vi "RC_Init.vi"(8 "error in (no error)":errorcluster, 10 "Condition #":i32, 11 "Reward_Condition in":refnum<class "Reward_Condition.lvclass">) -> (0 "error out":errorcluster, 3 "Reward_Condition out":refnum<class "Reward_Condition.lvclass">)   [LabVIEW 2018, in "Tracker.lvlib" / "Reward_Condition.lvclass"]
uses:
  Reward_Condition.lvclass
  Reward_SubCondition/Reward_SubCondition.lvclass
  Reward_Condition.lvclass/Reward_Condition.ctl
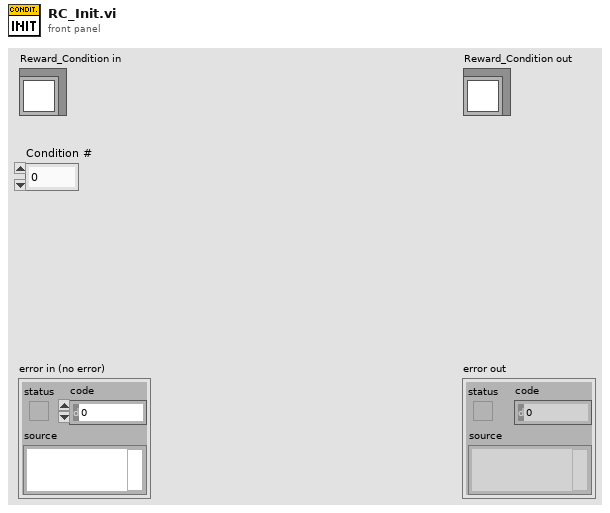
[diagram p1: front panel]
types:
  T1 = enum16{"None", "Port 1", "Port 2", "Port 3", "Port 4"}
  T2 = enum16{"None", "TTL pulse", "TTL trigger", "Air puff", "Liquid reward"}
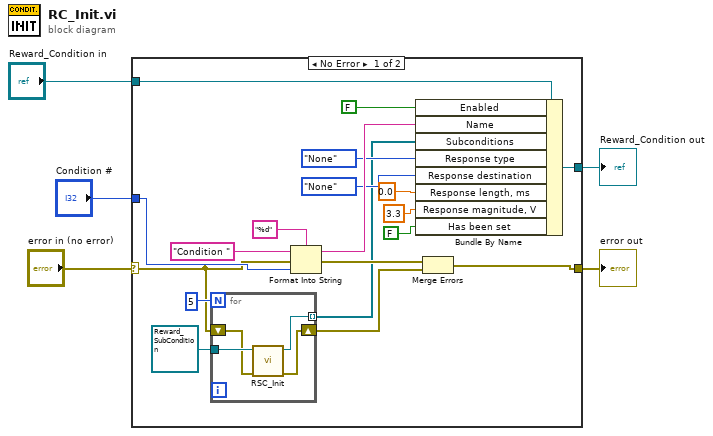
[diagram p0: block diagram]
diagram:
  n1 = case shown="No Error" "error in (no error)" {
    selector: "error in (no error)" -> [w8 w30]
    tunnel: [w7 w30] -> w4
    tunnel: [w23 w29] -> w2
    tunnel: "Reward_Condition in" -> [w24 w29]
    tunnel: "Condition #" -> [w20 _]
    frame No Error {
      n2 = for {
        N: 5 -> [_]
        tunnel: refnum<class "Reward_SubCondition.lvclass"> refnum ("Tracker.lvlib:Reward_SubCondition.lvclass") -> [w28]
        tunnel: [w27] -> w9 mode=indexing
        shift-right: [w25] -> w6
        shift-left: w8 -> [w26]
        n3 = call "RSC_Init.vi"("error in (no error)"=w26, "Reward_SubCondition in"=w28) -> ("error out"=w25:errorcluster, "Reward_SubCondition out"=w27:refnum<class "Reward_SubCondition.lvclass">)  [unwired: 8 in]
      }
      n4 = Format Into String(format string="%d", initial string="Condition ", error in=w8, w20) -> (resulting string=w19:string, error out=w13:errorcluster)
      n5 = Bundle By Name(cluster=w24, "Enabled"=FALSE, "Name"=w19, "Subconditions"=w9, "Response type"=T2."None", "Response destination"=T1."None", "Response length, ms"=0.0, "Response magnitude, V"=3.3, "Has been set"=FALSE) -> (w23:refnum<class "Reward_Condition.lvclass">)
      n6 = Merge Errors(w13, w6) -> (w7:errorcluster)
    }
    frame Error {
    }
  }
  "error out" <- w4
  "Reward_Condition out" <- w2
